vi "setFPGAReference.vi"(10 "FPGAReference":refnum<k20>, 11 "MyHealthAndStatusReadFIFO in":refnum<class "Accel1Channel1FIFO.lvclass">) -> (3 "MyHealthAndStatusReadFIFO out":refnum<class "Accel1Channel1FIFO.lvclass">)   [LabVIEW 2016, in "Accel1Channel1FIFO.lvclass"]
uses:
  Accel1Channel1FIFO.lvclass
  Accel1Channel1FIFO.lvclass/Accel1Channel1FIFO.ctl
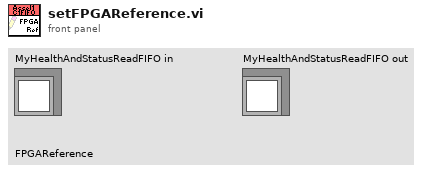
[diagram p1: front panel]
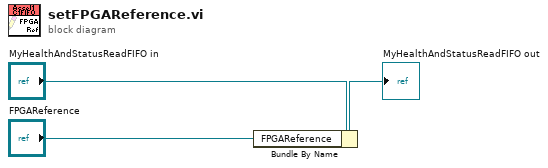
[diagram p0: block diagram]
diagram:
  n1 = Bundle By Name(cluster="MyHealthAndStatusReadFIFO in", "FPGAReference"="FPGAReference") -> (→"MyHealthAndStatusReadFIFO out":refnum<class "Accel1Channel1FIFO.lvclass">)
